vi "IntuitiveSteering_phi.vi"(0 "Input":dbl, 1 "Flap":dbl, 2 "Flap Saturation":dbl, 5 "Forward Time":dbl, 7 "Phase Shift":dbl, 9 "Max. Amplitude":dbl, 11 "nonZeroPositionIndex":i8, 12 "WhatDoesY":dbl, 13 "WhatDoesZ":dbl) -> (4 "Servo Position":T1)   [LabVIEW 2013]
uses:
  My Computer/Controls/Servo Position.ctl
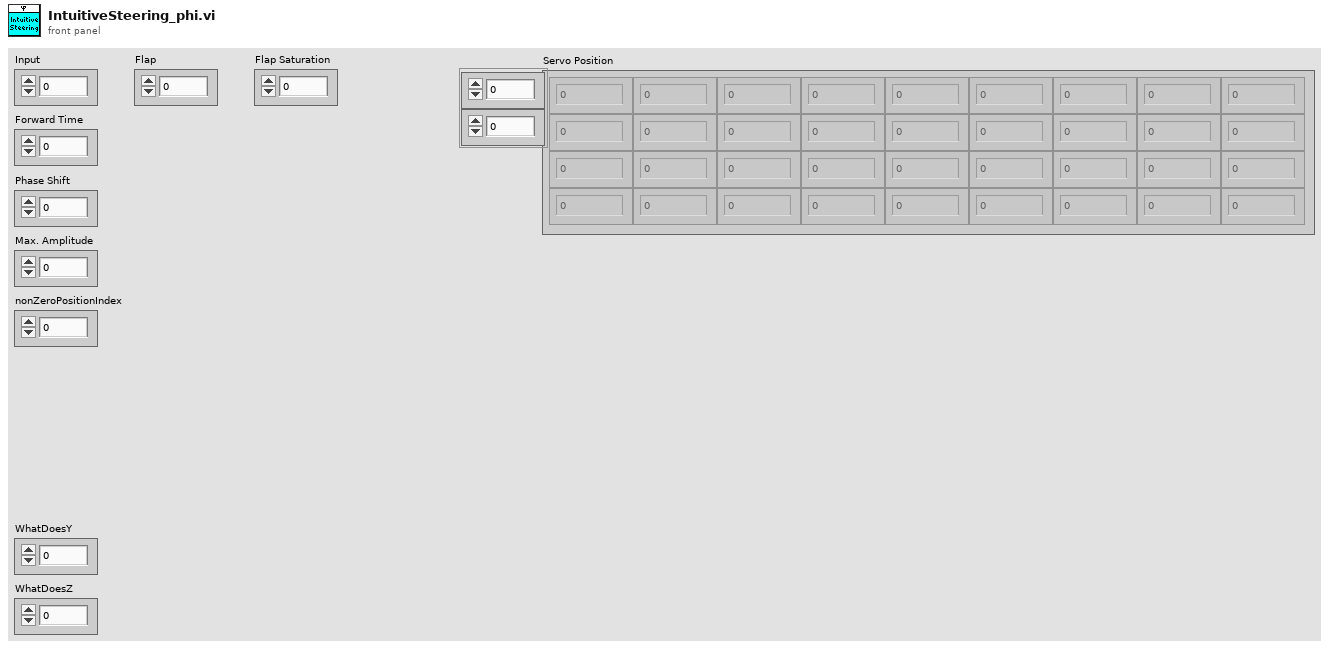
[diagram p1: front panel]
types:
  T1 = typedef "Servo Position.ctl" = dbl[][]
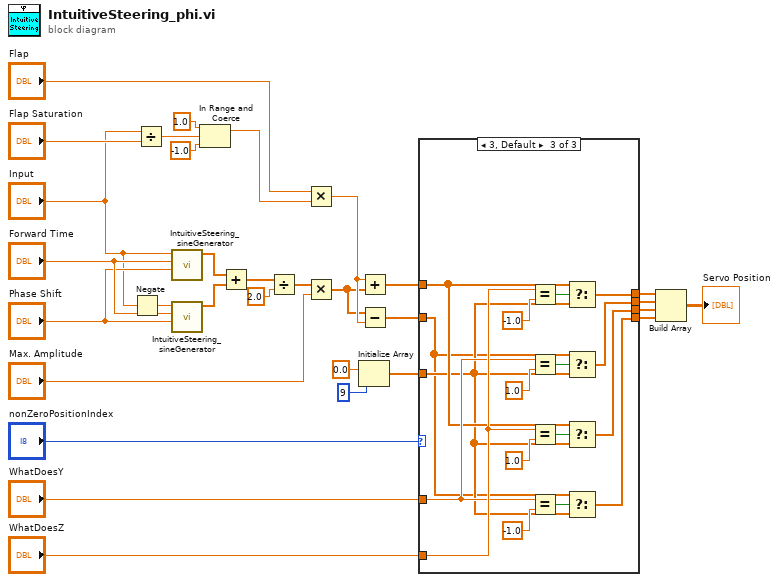
[diagram p0: block diagram]
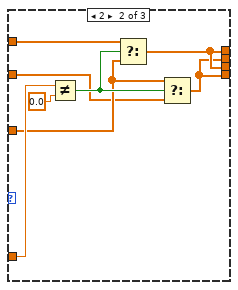
[diagram p3: hidden frame]
diagram:
  n1 = Negate(x="Input") -> (-x=w31:dbl)
  n2 = Divide(x="Input", y="Flap Saturation") -> (x/y=w5:dbl)
  n3 = call "IntuitiveSteering_sineGenerator.vi"("Phase Shift"="Phase Shift", "Forward Time"="Forward Time", "Input"="Input") -> ("Fin Position"=w29:dbl[])  [unwired: 8 in]
  n4 = call "IntuitiveSteering_sineGenerator.vi"("Phase Shift"="Phase Shift", "Forward Time"="Forward Time", "Input"=w31) -> ("Fin Position"=w28:dbl[])  [unwired: 8 in]
  n5 = In Range and Coerce(upper limit=1.0, x=w5, lower limit=-1.0) -> (coerced(x)=w6:dbl)  [unwired: 1 out]
  n6 = Add(x=w29, y=w28) -> (x+y=w26:dbl[])
  n7 = Divide(x=w26, y=2.0) -> (x/y=w16:dbl[])
  n8 = Multiply(x="Flap", y=w6) -> (x*y=w4:dbl)
  n9 = Multiply(x=w16, y="Max. Amplitude") -> (x*y=w3:dbl[])
  n10 = Initialize Array(0.0 ("element"), 9 ("dimension size")) -> (w12:dbl[])
  n11 = Add(x=w4, y=w3) -> (x+y=w17:dbl[])
  n12 = Subtract(x=w3, y=w4) -> (x-y=w2:dbl[])
  n13 = case shown="3, Default" "nonZeroPositionIndex" {
    tunnel: w17 -> [w33 w34 w45]
    tunnel: [w33 w38 w51] -> w24
    tunnel: [w32 w37 w50] -> w23
    tunnel: [w33 w38 w49] -> w22
    tunnel: [w32 w37 w44] -> w21
    tunnel: "WhatDoesY" -> [_ w41 w46]
    tunnel: "WhatDoesZ" -> [_ _ w53]
    tunnel: w12 -> [_ w36 w43]
    tunnel: w2 -> [w32 w35 w42]
    frame 1 {
    }
    frame 2 {
      n14 = Not Equal?(x=w41, y=0.0) -> (x != y?=w39:bool)
      n15 = Select(t=w34, s=w39, f=w36) -> (s? t:f=w38:dbl[])
      n16 = Select(t=w36, s=w39, f=w35) -> (s? t:f=w37:dbl[])
    }
    frame 3, Default {
      n17 = Equal?(x=w53, y=-1.0) -> (x = y?=w58:bool)
      n18 = Equal?(x=w46, y=1.0) -> (x = y?=w57:bool)
      n19 = Equal?(x=w53, y=1.0) -> (x = y?=w56:bool)
      n20 = Equal?(x=w46, y=-1.0) -> (x = y?=w47:bool)
      n21 = Select(t=w45, s=w58, f=w43) -> (s? t:f=w51:dbl[])
      n22 = Select(t=w42, s=w57, f=w43) -> (s? t:f=w50:dbl[])
      n23 = Select(t=w45, s=w56, f=w43) -> (s? t:f=w49:dbl[])
      n24 = Select(t=w42, s=w47, f=w43) -> (s? t:f=w44:dbl[])
    }
  }
  n25 = Build Array(w24, w23, w22, w21) -> (→"Servo Position":dbl[][])
